vi "CreateStringBufferOfDefinedSize.vi"(11 "size":i32) -> (2 "size (out)":i32, 3 "string":string)   [LabVIEW 2019]
doc: "Creates string buffer with defined size"
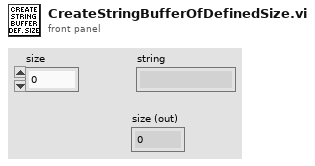
[diagram p1: front panel]
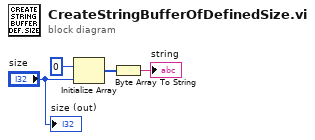
[diagram p0: block diagram]
diagram:
  n1 = Initialize Array(u8 0 ("element"), "size") -> (w3:u8[])
  n2 = Byte Array To String(unsigned byte array=w3) -> (string=→"string":string)
  "size (out)" <- "size"
